vi "UI Manual Operation.vi"(8 "error in (no error)":errorcluster) -> (0 "error out":errorcluster)   [LabVIEW 2019, in "UIs.lvlib"]
uses:
  UIs.lvlib
  TD Maunal Operation Page.ctl
panel:
  in  "Radio Buttons":T1
  in  "Back":bool
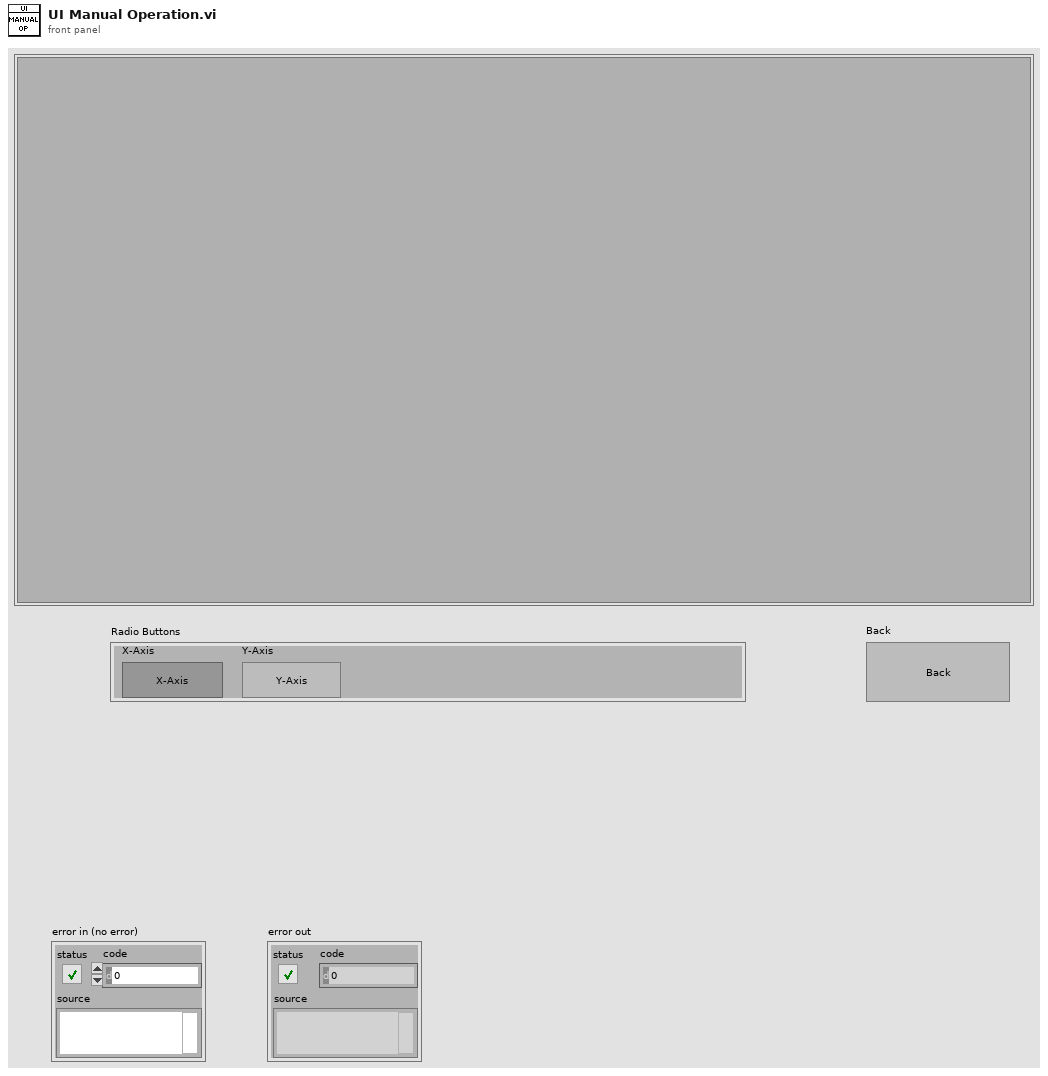
[diagram p1: front panel]
types:
  T1 = typedef "UIs.lvlib/TD Maunal Operation Page.ctl" = enum32{"X-Axis", "Y-Axis"}
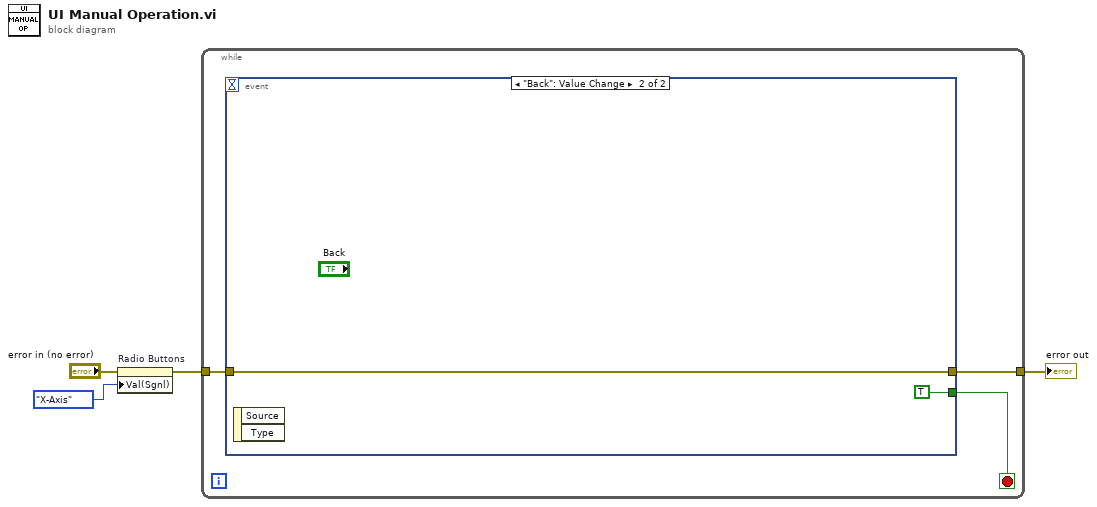
[diagram p0: block diagram]
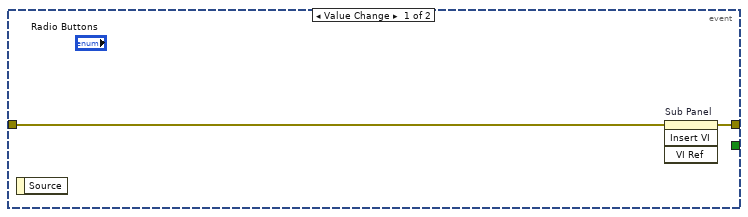
[diagram p2: hidden frame]
diagram:
  n1 = property on="Radio Buttons" class="RadioBtnsControl (strict)"(error in="error in (no error)", "Val(Sgnl)"=TD_Maunal_Operation_Page."X-Axis" ("Radio Buttons")) -> (error out=w1:errorcluster)  [unwired: 1 in, 1 out]
  n2 = while {
    tunnel: w1 -> [w7]
    tunnel: [w5] -> w4
    stop <- w6 stop-if-true
    n3 = event shown="[1] \"Back\": Value Change" {
      selector: _ -> [_ _]
      dyn-events: _ -> [_ _]
      timeout: _ -> [_ _]
      tunnel: w7 -> [w8 w10]
      tunnel: [_ TRUE] -> w6
      tunnel: [w9 w10] -> w5
      event Value Change {
        n4 = event-data() -> ()  [unwired: 1 in, 1 out]
        n5 = invoke on="Sub Panel" class="SubPnl" method="Insert VI"(error in=w8) -> (error out=w9:errorcluster)  [unwired: 3 in, 3 out]
      }
      event "Back": Value Change {
        n6 = event-data() -> ()  [unwired: 1 in, 2 out]
      }
    }
  }
  "error out" <- w4
